vi "Set Report Tab Width.vi"(4 "error in (no error)":errorcluster, 5 "measurement system (US)":u16(ring) items=["US", "Metric"], 6 "width (.25)":dbl=0.25 format="%.2f", 7 "report in":T1) -> (0 "error out":errorcluster, 3 "report out":T1)   [LabVIEW 2020]
doc: "Sets the tab width in the report."
uses:
  <vilib>/Utility/NIReport.llb/Generate Report Object Reference.ctl
  <vilib>/Utility/NIReport.llb/NI_report.lvclass
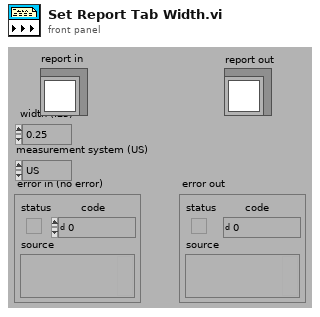
[diagram p1: front panel]
types:
  T1 = typedef "Generate Report Object Reference.ctl" = refnum<class "NI_report.lvclass">
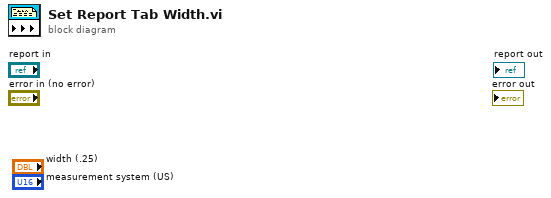
[diagram p0: block diagram]
diagram:
